vi "Read Std Dev.vi"(8 "error in (no error)":errorcluster, 11 "Std Dev in":refnum<class "Std Dev.lvclass">) -> (0 "error out":errorcluster, 1 "Channels w/ Std Dev":string[](array[string]), 2 "4 Data Points":dbl[](array[numeric]), 3 "Std Dev out":refnum<class "Std Dev.lvclass">)   [LabVIEW 2009, in "Std Dev.lvclass"]
doc: "Returns the Standard Deviation.\n\nPublic Interface for \"_Read.vi\""
uses:
  Std Dev.lvclass
  Std Dev.lvclass/Std Dev.ctl
  Readable/Readable.lvclass
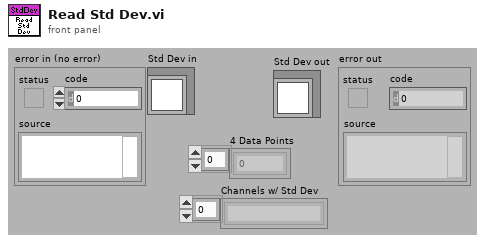
[diagram p1: front panel]
types:
  T1 = typedef "Readable.lvclass/Channel Names.ctl" = string[]
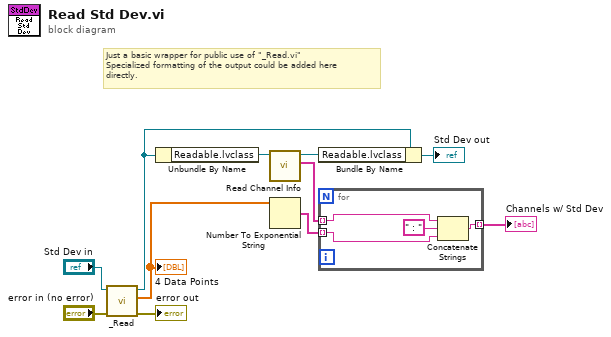
[diagram p0: block diagram]
diagram:
  # "Just a basic wrapper for public use of \"_Read.vi\"\nSpecialized formatting of the output could be added here\ndirectly."
  n1 = call-dynamic "_Read.vi"("error in (no error)"="error in (no error)", "Std Dev in"="Std Dev in") -> ("error out"=→"error out":errorcluster, "4 Data Points"=w9:dbl[], "Std Dev out"=w4:refnum<class "Std Dev.lvclass">)  [unwired: 7 in]
  "4 Data Points" <- w9
  n2 = Unbundle By Name(w4) -> ("Readable.lvclass"=w7:refnum<class "Readable.lvclass">)
  n3 = call "Read Channel Info.vi"("Readable.lvclass in"=w7) -> ("Channel Names"=w1:T1, "Readable.lvclass out"=w6:refnum<class "Readable.lvclass">)  [unwired: 6 in, 3 out]
  n4 = Number To Exponential String(number=w9) -> (E-format string=w3:string[])  [unwired: 3 in]
  n5 = Bundle By Name(cluster=w4, "Readable.lvclass"=w6) -> (→"Std Dev out":refnum<class "Std Dev.lvclass">)
  n6 = for {
    tunnel: w3 -> [w13] mode=indexing
    tunnel: w1 -> [w14] mode=indexing
    tunnel: [w15] -> w2 mode=indexing
    n7 = Concatenate Strings(w14, " : " ("string"), w13) -> (w15:string)
  }
  "Channels w/ Std Dev" <- w2
